vi "2D FFT of a Pulse.vi"() -> ()   [LabVIEW 2023]
doc: "This example demonstrates how to use the FFT VIs to compute the two-dimensional FFT, using a simple rectangular step function within a square image as the original 2D image to transform. It also has other kind of inputs to demonstrate how this would impact the 2D image."
uses:
  <vilib>/Analysis/baseanly.llb/Real Outer Product.vi
  <vilib>/Analysis/2dsp.llb/2D Real FFT.vi
  <vilib>/Analysis/2dsp.llb/2D Inverse Real FFT.vi
  <vilib>/Analysis/1siggen.llb/General Aperiodic Triangle.vi
  <vilib>/Analysis/1siggen.llb/General Gaussian Monopulse.vi
  <vilib>/Analysis/NI_AALPro.lvlib
  <vilib>/Analysis/NI_AALBase.lvlib
panel:
  in  "asymmetry x for triangle":dbl(slide)=0.5 step=0.1 scale=0.0..1.0
  in  "asymmetry y for triangle":dbl(slide)=0.5 step=0.1 scale=0.0..1.0
  in  "shift?":bool=TRUE
  in  "Stop":bool
  in  "Type of image":u16(ring) items=["Pulse", "Triangle", "Noise", "Sine"]
  in  "amplitude":dbl(slide)=100.0 scale=0.0..200.0
  out "Inverse 2DFFT":dbl[][](graph)
  out "2DFFT{Image}":dbl[][](graph)
  out "Image":dbl[][](graph)
  # "Overview: This VI demonstrates how to decompose and recompose images with the FFT VI and Inverse FFT VI.\nRequirement: LabVIEW Full Development System\nInstructions:\n1. Run the VI.\n2. Change the Type of image and amplitude to study how the FFT behaves.\n3. Change the cursor position of the Image to verify how the frequency response changes as you change the size of the image.\n4. Click Stop to stop the VI."
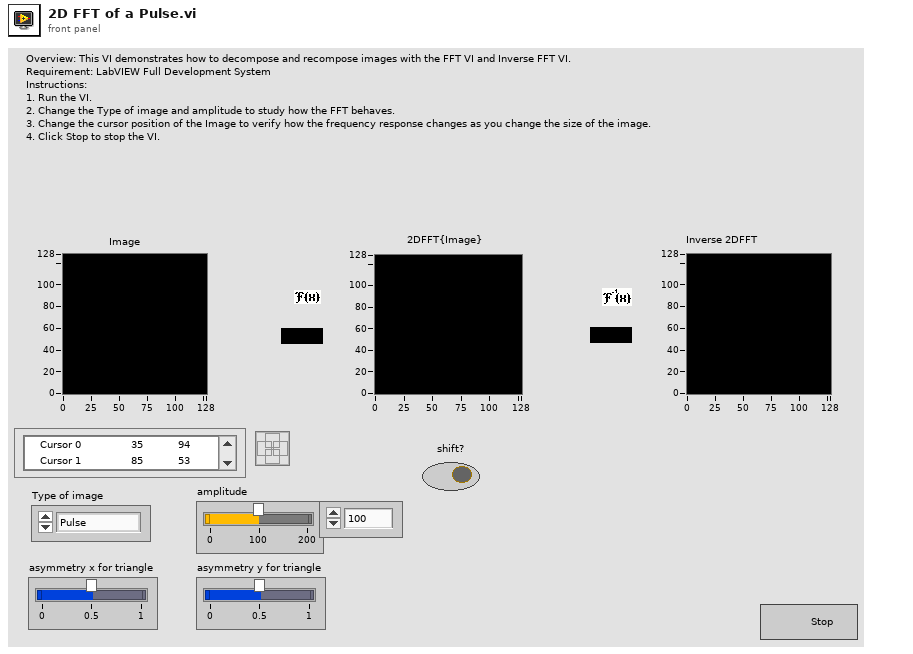
[diagram p1: front panel]
types:
  T1 = typedef "NI_Matrix.lvlib/RealMatrix.ctl" = dbl[][]
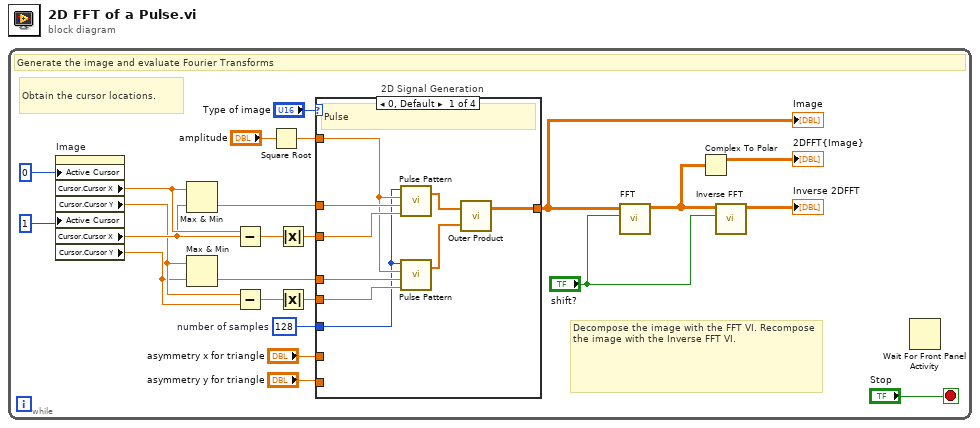
[diagram p0: block diagram]
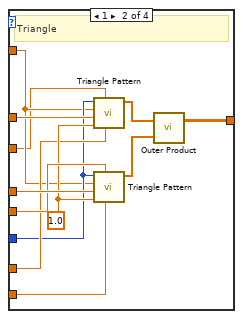
[diagram p2: hidden frame]
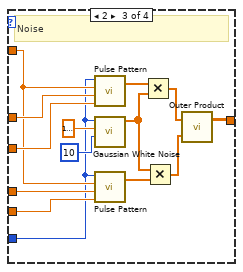
[diagram p3: hidden frame]
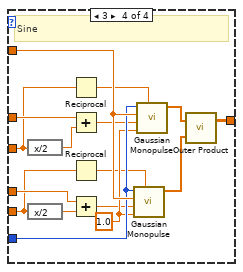
[diagram p4: hidden frame]
diagram:
  n1 = while {
    stop <- "Stop" stop-if-true
    w2 = 128  # number of samples
    # "Decompose the image with the FFT VI. Recompose the image with the Inverse FFT VI."
    # "Obtain the cursor locations."
    # "Generate the image and evaluate Fourier Transforms"
    n2 = property on="Image" class="IntGraph (strict)"("Active Cursor"=u32 0, "Active Cursor"=u32 1) -> ("Cursor.Cursor X"=w15:dbl, "Cursor.Cursor Y"=w10:dbl, "Cursor.Cursor X"=w14:dbl, "Cursor.Cursor Y"=w9:dbl)  [unwired: 2 in, 2 out]
    n3 = Max & Min(x=w15, y=w14) -> (min(x,y)=w17:dbl)  [unwired: 1 out]
    n4 = Max & Min(x=w10, y=w9) -> (min(x,y)=w16:dbl)  [unwired: 1 out]
    n5 = Subtract(x=w15, y=w14) -> (x-y=w13:dbl)
    n6 = Subtract(x=w10, y=w9) -> (x-y=w11:dbl)
    n7 = Square Root(x="amplitude") -> (sqrt(x)=w1:dbl)
    n8 = Absolute Value(x=w13) -> (abs(x)=w12:dbl)
    n9 = Absolute Value(x=w11) -> (abs(x)=w8:dbl)
    n10 = case "2D Signal Generation" shown="0, Default" "Type of image" {
      tunnel: [w31 w45 w57 w73] -> w23
      tunnel: w17 -> [w30 w44 w56 w69]
      tunnel: w12 -> [w29 w34 w55 w62]
      tunnel: w16 -> [w28 w43 w54 w67]
      tunnel: w8 -> [w27 w42 w53 w60]
      tunnel: w1 -> [w26 w37 w52 w72]
      tunnel: "asymmetry y for triangle" -> [_ w40 _ _]
      tunnel: "asymmetry x for triangle" -> [_ w39 _ _]
      tunnel: w2 -> [w25 w38 w46 w71]
      frame 0, Default {
        # "Pulse"
        n11 = call <vilib>:"Pulse Pattern.vi"("width"=w29, "delay"=w30, "amplitude"=w26, "samples"=w25) -> ("Pulse Pattern"=w33:dbl[])  [unwired: 1 out]
        n12 = call <vilib>:"Pulse Pattern.vi"("width"=w27, "delay"=w28, "amplitude"=w26, "samples"=w25) -> ("Pulse Pattern"=w32:dbl[])  [unwired: 1 out]
        n13 = call-poly <vilib>:"Outer Product.vi"("Y Vector"=w32, "X Vector"=w33) -> ("Outer Product"=w31:T1)  [unwired: 1 out]
      }
      frame 1 {
        w41 = 1.0 ("delta t (s)")
        # "Triangle"
        n14 = call <vilib>:"Triangle Pattern.vi"("asymmetry"=w39, "width (s)"=w34, "delta t (s)"=w41, "delay (s)"=w44, "amplitude"=w37, "samples"=w38) -> ("Triangle Pattern"=w35:dbl[])  [unwired: 4 in, 1 out]
        n15 = call <vilib>:"Triangle Pattern.vi"("asymmetry"=w40, "width (s)"=w42, "delta t (s)"=w41, "delay (s)"=w43, "amplitude"=w37, "samples"=w38) -> ("Triangle Pattern"=w36:dbl[])  [unwired: 4 in, 1 out]
        n16 = call-poly <vilib>:"Outer Product.vi"("Y Vector"=w36, "X Vector"=w35) -> ("Outer Product"=w45:T1)  [unwired: 1 out]
      }
      frame 2 {
        # "Noise"
        n17 = call <vilib>:"Pulse Pattern.vi"("width"=w55, "delay"=w56, "amplitude"=w52, "samples"=w46) -> ("Pulse Pattern"=w59:dbl[])  [unwired: 1 out]
        n18 = call <vilib>:"Gaussian White Noise.vi"("seed"=10, "standard deviation"=1.0000000000000002, "samples"=w46) -> ("Gaussian noise pattern"=w48:dbl[])  [unwired: 7 in, 1 out]
        n19 = call <vilib>:"Pulse Pattern.vi"("width"=w53, "delay"=w54, "amplitude"=w52, "samples"=w46) -> ("Pulse Pattern"=w58:dbl[])  [unwired: 1 out]
        n20 = Multiply(x=w59, y=w48) -> (x*y=w51:dbl[])
        n21 = Multiply(x=w48, y=w58) -> (x*y=w49:dbl[])
        n22 = call-poly <vilib>:"Outer Product.vi"("Y Vector"=w49, "X Vector"=w51) -> ("Outer Product"=w57:T1)  [unwired: 1 out]
      }
      frame 3 {
        w70 = 1.0 ("delta t (s)")
        # "Sine"
        n23 = expression code="x/2"(w62) -> (w63:dbl)
        n24 = expression code="x/2"(w60) -> (w65:dbl)
        n25 = Reciprocal(x=w62) -> (1/x=w64:dbl)
        n26 = Add(x=w69, y=w63) -> (x+y=w68:dbl)
        n27 = Reciprocal(x=w60) -> (1/x=w61:dbl)
        n28 = Add(x=w67, y=w65) -> (x+y=w66:dbl)
        n29 = call <vilib>:"Gaussian Monopulse.vi"("center frequency (Hz)"=w61, "delta t (s)"=w70, "delay (s)"=w66, "amplitude"=w72, "samples"=w71) -> ("Gaussian Monopulse"=w74:dbl[])  [unwired: 5 in, 1 out]
        n30 = call <vilib>:"Gaussian Monopulse.vi"("center frequency (Hz)"=w64, "delta t (s)"=w70, "delay (s)"=w68, "amplitude"=w72, "samples"=w71) -> ("Gaussian Monopulse"=w75:dbl[])  [unwired: 5 in, 1 out]
        n31 = call-poly <vilib>:"Outer Product.vi"("Y Vector"=w74, "X Vector"=w75) -> ("Outer Product"=w73:T1)  [unwired: 1 out]
      }
    }
    "Image" <- w23
    n32 = call-poly <vilib>:"FFT.vi"("shift?"="shift?", "X"=w23) -> ("FFT {X}"=w6:cdb[][])  [unwired: 8 in, 1 out]
    n33 = Complex To Polar(r * e^(i*theta)=w6) -> (r=→"2DFFT{Image}":dbl[][])  [unwired: 1 out]
    n34 = call-poly <vilib>:"Inverse FFT.vi"("shift?"="shift?", "FFT {X}"=w6) -> ("X"=→"Inverse 2DFFT":dbl[][])  [unwired: 8 in, 1 out]
    n35 = Wait For Front Panel Activity() -> ()  [unwired: 3 in, 1 out]
  }
